vi "Overlay Line with Arrows.vi"(6 "Color":u32(colorbox), 7 "Draw line?":bool=TRUE, 8 "error in (no error)":errorcluster, 9 "Arrows":cluster{"Start point":bool, "End point":bool}, 10 "Line Coordinates":T1 {"Point2"."Y" format="%.2f"; "Point2"."X" format="%.2f"; "Point1"."Y" format="%.2f"; "Point1"."X" format="%.2f"}, 11 "Image In":T2) -> (0 "error out":errorcluster, 3 "Image Out":T2)   [LabVIEW 2015]
uses:
  <vilib>/vision/Image Controls.llb/IMAQ Image.ctl
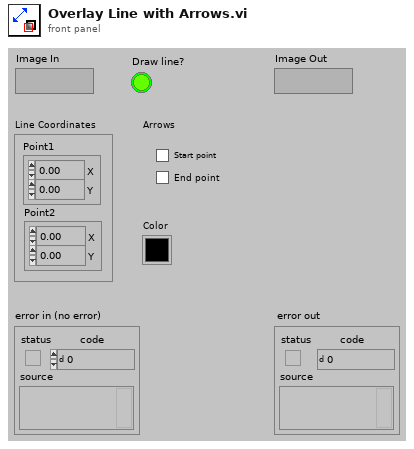
[diagram p1: front panel]
types:
  T1 = cluster{"Point1":cluster{"X":sgl, "Y":sgl}, "Point2":cluster{"X":sgl, "Y":sgl}}
  T2 = typedef "IMAQ Image.ctl" = refnum<image>
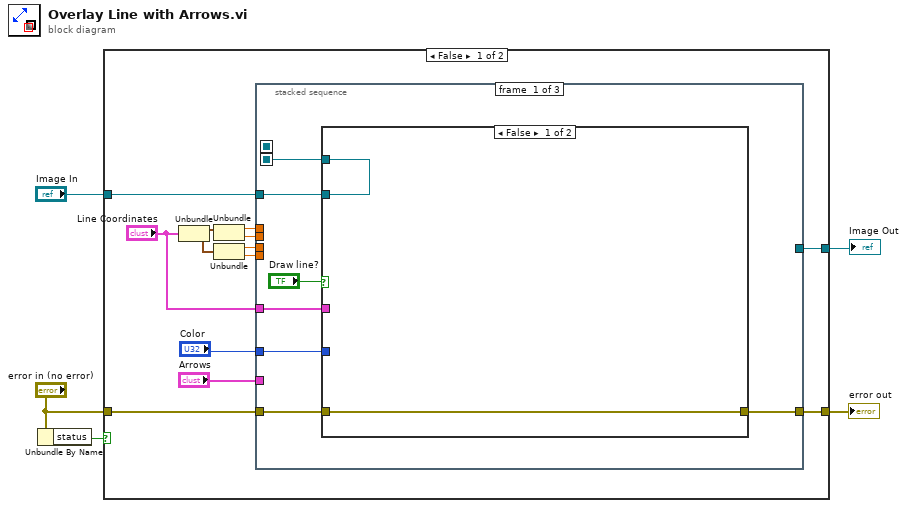
[diagram p0: block diagram]
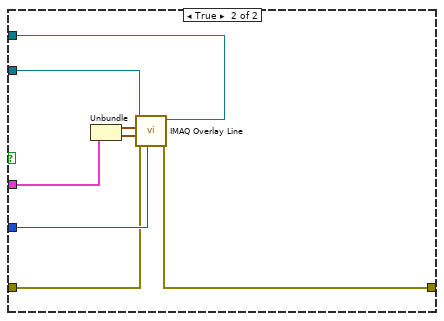
[diagram p2: hidden frame]
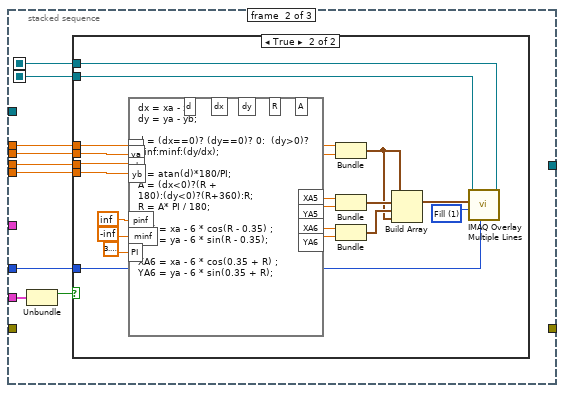
[diagram p3: hidden frame]
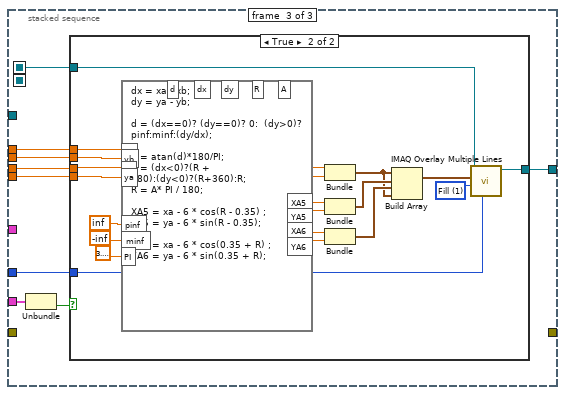
[diagram p5: hidden frame]
diagram:
  n1 = Unbundle By Name("error in (no error)") -> ("status"=w3:bool)
  n2 = case shown="False" w3 {
    tunnel: "Image In" -> [w9 w94]
    tunnel: [w8 w94] -> w4
    tunnel: [w6 w95] -> w2
    tunnel: "error in (no error)" -> [w7 w95]
    frame False {
      n3 = Unbundle("Line Coordinates") -> ("Point1"=w13:cluster{"X":sgl, "Y":sgl}, "Point2"=w12:cluster{"X":sgl, "Y":sgl})
      n4 = Unbundle(w13) -> ("X"=w17:sgl, "Y"=w16:sgl)
      n5 = Unbundle(w12) -> ("X"=w15:sgl, "Y"=w14:sgl)
      n6 = stacked-sequence {
        seq-local: [w25 _ _] -> [_ w38 _]
        seq-local: [_ w37 _] -> [_ _ w67]
        tunnel: "Arrows" -> [_ w44 w73]
        tunnel: w17 -> [_ w43 w72]
        tunnel: w16 -> [_ w42 w71]
        tunnel: w15 -> [_ w41 w70]
        tunnel: w14 -> [_ w40 w69]
        tunnel: "Line Coordinates" -> [w23 _ _]
        tunnel: "Color" -> [w24 w36 w66]
        tunnel: w9 -> [w22 _ _]
        tunnel: [_ _ w65] -> w8
        tunnel: w7 -> [w21 _ _]
        tunnel: [w20 _ _] -> w6
        frame #0 {
          n7 = case shown="False" "Draw line?" {
            tunnel: [w27 w35] -> w25
            tunnel: w24 -> [_ w34]
            tunnel: w23 -> [_ w33]
            tunnel: w22 -> [w27 w30]
            tunnel: w21 -> [w26 w29]
            tunnel: [w26 w28] -> w20
            frame False {
            }
            frame True {
              n8 = Unbundle(w33) -> ("Point1"=w32:cluster{"X":sgl, "Y":sgl}, "Point2"=w31:cluster{"X":sgl, "Y":sgl})
              n9 = call "IMAQ Overlay Line"("Color"=w34, "error in (no error)"=w29, "End Point"=w31, "Start Point"=w32, "Image"=w30) -> ("error out"=w28:errorcluster, "Image Out"=w35:T2)  [unwired: 1 in, 4 out]
            }
          }
        }
        frame #1 {
          n10 = Unbundle(w44) -> ("Start point"=w39:bool)  [unwired: 1 out]
          n11 = case shown="True" w39 {
            tunnel: w43 -> [_ w53]
            tunnel: w42 -> [_ w52]
            tunnel: w41 -> [_ w54]
            tunnel: w40 -> [_ w51]
            tunnel: w38 -> [w45 w50]
            tunnel: [w45 w48] -> w37
            tunnel: w36 -> [_ w47]
            frame False {
            }
            frame True {
              w46 = u32 1 items=["Frame", "Fill"] ("Drawing Mode (Frame)")
              n12 = formula code="dx = xa - xb;\ndy = ya - yb;\n\nd = (dx==0)? (dy==0)? 0:  (dy>0)? pinf:minf:(dy/dx);\n\nR = atan(d)*180/PI;\nA = (dx<0)?(R + 180):(dy<0)?(R+360):R;\nR = A* PI / 180;\n\nXA5 = xa - 6 * cos(R - 0.35) ;\nYA5 = ya - 6 * sin(R - 0.35);\n\nXA6 = xa - 6 * cos(0.35 + R) ;\nYA6 = ya - 6 * sin(0.35 + R);"("xa"=w53, "ya"=w52, "xb"=w54, "yb"=w51, "pinf"=inf, "minf"=-inf, "PI"=3.141592653589793) -> ("XA5"=w61:dbl, "YA5"=w60:dbl, "XA6"=w59:dbl, "YA6"=w58:dbl)  [unwired: 5 out]
              n13 = Bundle("X"=w53, "Y"=w52) -> (w55:cluster{"X":sgl, "Y":sgl})  [unwired: 1 out]
              n14 = Bundle("XA5"=w61, "YA5"=w60) -> (w57:cluster{"XA5":dbl, "YA5":dbl})  [unwired: 1 out]
              n15 = Bundle("XA6"=w59, "YA6"=w58) -> (w56:cluster{"XA6":dbl, "YA6":dbl})  [unwired: 1 out]
              n16 = Build Array(w55, w57, w56, w55) -> (w49:cluster{"XA6":dbl, "YA6":dbl}[])
              n17 = call "IMAQ Overlay Multiple Lines"("Color"=w47, "Drawing Mode (Frame)"=w46, "Line End Points"=w49, "Image"=w50) -> ("Image Out"=w48:T2)  [unwired: 2 in, 5 out]
            }
          }
        }
        frame #2 {
          n18 = Unbundle(w73) -> ("End point"=w68:bool)  [unwired: 1 out]
          n19 = case shown="True" w68 {
            tunnel: w72 -> [_ w90]
            tunnel: w71 -> [_ w89]
            tunnel: w70 -> [_ w88]
            tunnel: w69 -> [_ w87]
            tunnel: w67 -> [w74 w78]
            tunnel: [w74 w77] -> w65
            tunnel: w66 -> [_ w76]
            frame False {
            }
            frame True {
              w75 = u32 1 items=["Frame", "Fill"] ("Drawing Mode (Frame)")
              n20 = formula code="dx = xa - xb;\ndy = ya - yb;\n\nd = (dx==0)? (dy==0)? 0:  (dy>0)? pinf:minf:(dy/dx);\n\nR = atan(d)*180/PI;\nA = (dx<0)?(R + 180):(dy<0)?(R+360):R;\nR = A* PI / 180;\n\nXA5 = xa - 6 * cos(R - 0.35) ;\nYA5 = ya - 6 * sin(R - 0.35);\n\nXA6 = xa - 6 * cos(0.35 + R) ;\nYA6 = ya - 6 * sin(0.35 + R);"("xb"=w90, "yb"=w89, "xa"=w88, "ya"=w87, "pinf"=inf, "minf"=-inf, "PI"=3.141592653589793) -> ("XA5"=w86:dbl, "YA5"=w85:dbl, "XA6"=w84:dbl, "YA6"=w83:dbl)  [unwired: 5 out]
              n21 = Bundle("X"=w88, "Y"=w87) -> (w80:cluster{"X":sgl, "Y":sgl})  [unwired: 1 out]
              n22 = Bundle("XA5"=w86, "YA5"=w85) -> (w82:cluster{"XA5":dbl, "YA5":dbl})  [unwired: 1 out]
              n23 = Bundle("XA6"=w84, "YA6"=w83) -> (w81:cluster{"XA6":dbl, "YA6":dbl})  [unwired: 1 out]
              n24 = Build Array(w80, w82, w81, w80) -> (w79:cluster{"XA6":dbl, "YA6":dbl}[])
              n25 = call "IMAQ Overlay Multiple Lines"("Color"=w76, "Drawing Mode (Frame)"=w75, "Line End Points"=w79, "Image"=w78) -> ("Image Out"=w77:T2)  [unwired: 2 in, 5 out]
            }
          }
        }
      }
    }
    frame True {
    }
  }
  "error out" <- w2
  "Image Out" <- w4
